vi "WPI_CANJaguar_ClearAck.vi"(8 "DevStatus":errorcluster, 11 "Device Number":u8) -> (0 "error out":errorcluster)   [LabVIEW 2016]
uses:
  <vilib>/Rock Robotics/WPI/CAN/Jaguar/SubVIs/WPI_CAN_MotorMessageIDs.ctl
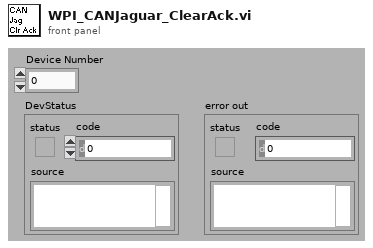
[diagram p1: front panel]
types:
  T1 = typedef "WPI_CAN_MotorMessageIDs.ctl" = u32
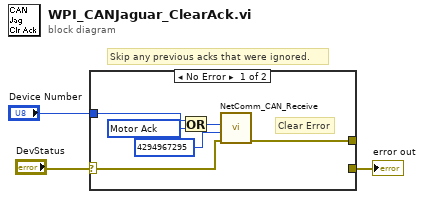
[diagram p0: block diagram]
diagram:
  # "Skip any previous acks that were ignored."
  n1 = case shown="No Error" "DevStatus" {
    selector: "DevStatus" -> [w5 w10]
    tunnel: [_ w10] -> w3
    tunnel: "Device Number" -> [w9 _]
    tunnel: [w4 _] -> _
    frame No Error {
      w7 = T1 33693696 items=["Volt Enable"=33685504, "Volt Disable"=33685568, "Volt Set"=33685632, "Volt Set Ramp"=33685696, "Volt Set No Ack"=33686080, "Speed Enable"=33686528, "Speed Disable"=33686592, "Speed Set"=33686656, "Speed P"=33686720, "Speed I"=33686784, "Speed D"=33686848, "Speed Ref"=33686912, "Speed Set No Ack"=33687232, "Volt Comp Enable"=33687552, "Volt Comp Disable"=33687616, "Volt Comp Set"=33687680, "Volt Comp In Ramp"=33687744, "Volt Comp Comp Ramp"=33687808, "Volt Comp Set No Ack"=33688128, "Position Enable"=33688576, "Position Disable"=33688640, "Position Set"=33688704, "Position P"=33688768, "Position I"=33688832, "Position D"=33688896, "Position Ref"=33688960, "Position Set No Ack"=33689280, "Current Enable"=33689600, "Current Disable"=33689664, "Current Set"=33689728, "Current P"=33689792, "Current I"=33689856, "Current D"=33689920, "Current Set No Ack"=33690240, "Status Percent VBus"=33690624, "Status VBus"=33690688, "Status Current"=33690752, "Status Temp"=33690816, "Status Position"=33690880, "Status Speed"=33690944, "Status Limit"=33691008, "Status Fault"=33691072, "Status Power"=33691136, "Status Control Mode"=33691200, "Status VOut"=33691264, "Status Sticky Fault"=33691328, "Status Fault Count"=33691392, "Periodic Status Enable 0"=33691648, "Periodic Status Enable 1"=33691712, "Periodic Status Enable 2"=33691776, "Periodic Status Enable 3"=33691840, "Periodic Status Config 0"=33691904, "Periodic Status Config 1"=33691968, "Periodic Status Config 2"=33692032, "Periodic Status Config 3"=33692096, "Periodic Status Data 0"=33692160, "Periodic Status Data 1"=33692224, "Periodic Status Data 2"=33692288, "Periodic Status Data 3"=33692352, "Config Num Brushes"=33692672, "Config Encoder Lines"=33692736, "Config Pot Turns"=33692800, "Config Brake Coast"=33692864, "Config Limit Mode"=33692928, "Config Limit Fwd"=33692992, "Config Limit Rev"=33693056, "Config Max VOut"=33693120, "Config Fault Time"=33693184, "Motor Ack"=33693696] ("CAN Motor Message IDs")
      # "Clear Error"
      n2 = Or(x=w9, y=w7) -> (x .or. y?=w6:T1)
      n3 = call <vilib>:"NetComm_CAN_Receive.vi"("error in (no error)"=w5, "Message ID Mask"=u32 4294967295 ("timeoutMs"), "Message ID"=w6) -> ("error out"=w4:errorcluster)  [unwired: 8 out]
    }
    frame Error {
    }
  }
  "error out" <- w3
